vi "Unlock Publication.vi"(6 "Publisher ID":string, 8 "error in (no error)":errorcluster, 9 "Datum Type":variant, 10 "Datum Name":string, 11 "IMediator In":refnum<class "IMediator.lvclass">) -> (0 "error out":errorcluster, 3 "IMediator Out":refnum<class "IMediator.lvclass">)   [LabVIEW 2018, in "MVA Framework.lvlib" / "IMediator.lvlib" / "IMediator.lvclass"]
doc: "抽象方法\n解锁发布者"
uses:
  IMediator.lvclass
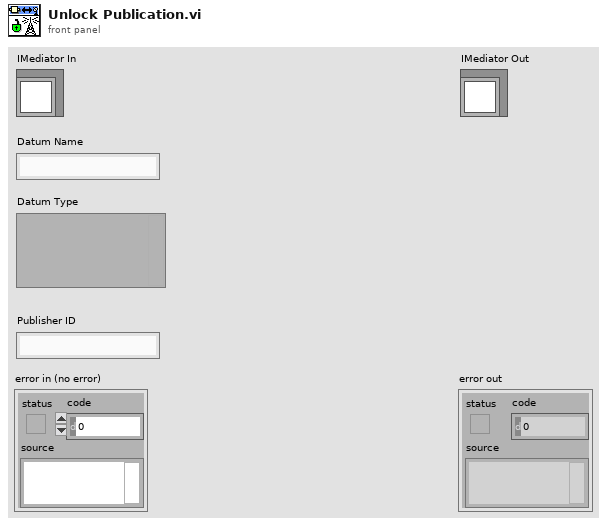
[diagram p1: front panel]
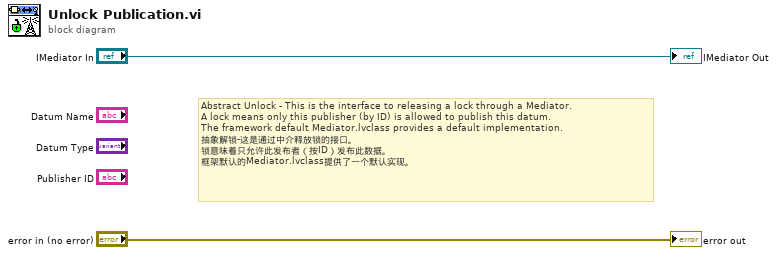
[diagram p0: block diagram]
diagram:
  # "Abstract Unlock - This is the interface to releasing a lock through a Mediator.\nA lock means only this publisher (by ID) is allowed to publish this datum.\nThe framework default Mediator.lvclass provides a default implementation.\n抽象解锁-这是通过中介释放锁的接口。\n锁意味着只允许此发布者（按ID）发布此数据。\n框架默认的Mediator.lvclass提供了一个默认实现。"
  "error out" <- "error in (no error)"
  "IMediator Out" <- "IMediator In"
